vi "ConversioneDati.vi"(4 "Stato Conversione":enum16{"CONVERTI_IN", "CONVERTI_OUT"}(ring), 10 "Data":dbl, 11 "Impostazioni Conversione":string[](array[string])) -> (3 "Dato Convertito":dbl)   [LabVIEW 2016]
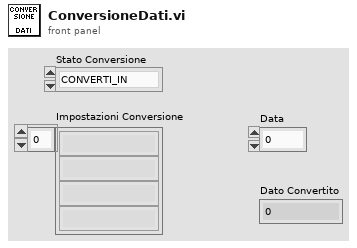
[diagram p1: front panel]
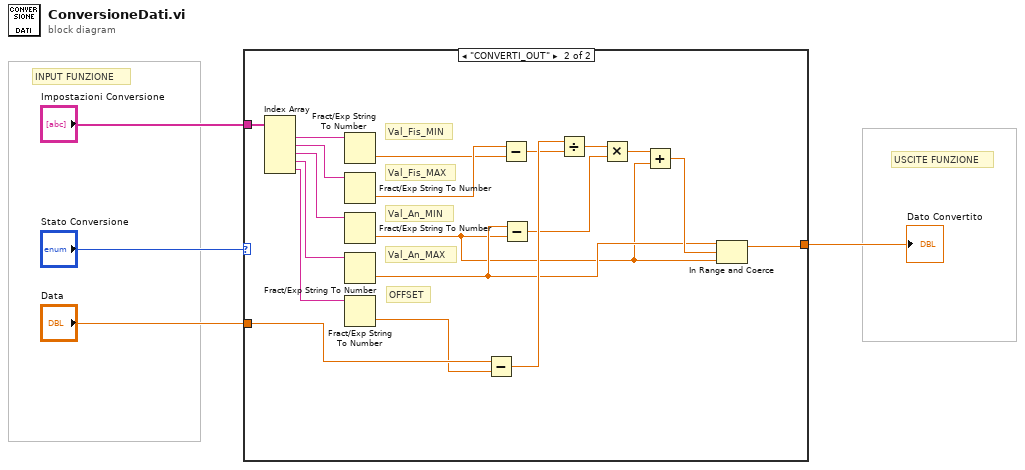
[diagram p0: block diagram]
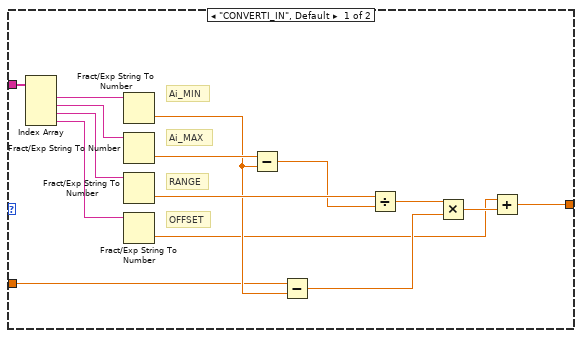
[diagram p2: hidden frame]
diagram:
  # "USCITE FUNZIONE"
  # "INPUT FUNZIONE"
  n1 = case shown="\"CONVERTI_OUT\"" "Stato Conversione" {
    tunnel: "Impostazioni Conversione" -> [w19 w34]
    tunnel: [w9 w30] -> w3
    tunnel: "Data" -> [w5 w32]
    frame "CONVERTI_IN", Default {
      # "OFFSET"
      # "RANGE"
      # "Ai_MAX"
      # "Ai_MIN"
      n2 = Index Array(array=w19) -> (element #1=w18:string, element #2=w8:string, element #3=w7:string, element #4=w6:string)  [unwired: 4 in]
      n3 = Fract/Exp String To Number(string=w18) -> (number=w14:dbl)  [unwired: 3 in, 1 out]
      n4 = Fract/Exp String To Number(string=w8) -> (number=w16:dbl)  [unwired: 3 in, 1 out]
      n5 = Fract/Exp String To Number(string=w7) -> (number=w17:dbl)  [unwired: 3 in, 1 out]
      n6 = Fract/Exp String To Number(string=w6) -> (number=w10:dbl)  [unwired: 3 in, 1 out]
      n7 = Subtract(x=w16, y=w14) -> (x-y=w15:dbl)
      n8 = Subtract(x=w5, y=w14) -> (x-y=w12:dbl)
      n9 = Divide(x=w17, y=w15) -> (x/y=w13:dbl)
      n10 = Multiply(x=w13, y=w12) -> (x*y=w11:dbl)
      n11 = Add(x=w10, y=w11) -> (x+y=w9:dbl)
    }
    frame "CONVERTI_OUT" {
      # "OFFSET"
      # "Val_An_MAX"
      # "Val_An_MIN"
      # "Val_Fis_MAX"
      # "Val_Fis_MIN"
      n12 = Index Array(array=w34) -> (element #1=w38:string, element #2=w37:string, element #3=w36:string, element #4=w35:string, element #5=w33:string)  [unwired: 5 in]
      n13 = Fract/Exp String To Number(string=w38) -> (number=w28:dbl)  [unwired: 3 in, 1 out]
      n14 = Fract/Exp String To Number(string=w37) -> (number=w29:dbl)  [unwired: 3 in, 1 out]
      n15 = Fract/Exp String To Number(string=w36) -> (number=w20:dbl)  [unwired: 3 in, 1 out]
      n16 = Fract/Exp String To Number(string=w35) -> (number=w21:dbl)  [unwired: 3 in, 1 out]
      n17 = Fract/Exp String To Number(string=w33) -> (number=w31:dbl)  [unwired: 3 in, 1 out]
      n18 = Subtract(x=w32, y=w31) -> (x-y=w27:dbl)
      n19 = Subtract(x=w29, y=w28) -> (x-y=w26:dbl)
      n20 = Subtract(x=w21, y=w20) -> (x-y=w22:dbl)
      n21 = Divide(x=w27, y=w26) -> (x/y=w25:dbl)
      n22 = Multiply(x=w25, y=w22) -> (x*y=w24:dbl)
      n23 = Add(x=w24, y=w20) -> (x+y=w23:dbl)
      n24 = In Range and Coerce(upper limit=w21, x=w23, lower limit=w20) -> (coerced(x)=w30:dbl)  [unwired: 1 out]
    }
  }
  "Dato Convertito" <- w3
